vi "create harp files (main).vi"() -> ()   [LabVIEW 2010]
panel:
  in  "Close":bool
  in  "Create":bool
  in  "Create these ones?":bool
  in  "path":path
  # "Files that can be updated through this script\nwithout affecting the application code:\n - main.c\n - app.h\n - app_funcs.h\n - app_ios_and_regs.h\n - app_ios_and_regs.c"
  # "Files to give extra caution:\n - app.c\n - app_funcs.c\n - interrupts.c"
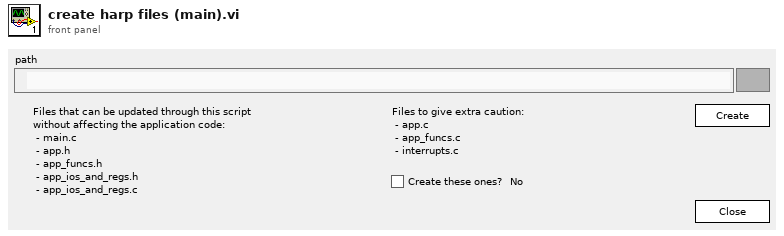
[diagram p1: front panel]
types:
  T1 = enum16{"open", "replace", "create", "open or create", "replace or create", "replace or create with confirmation"}
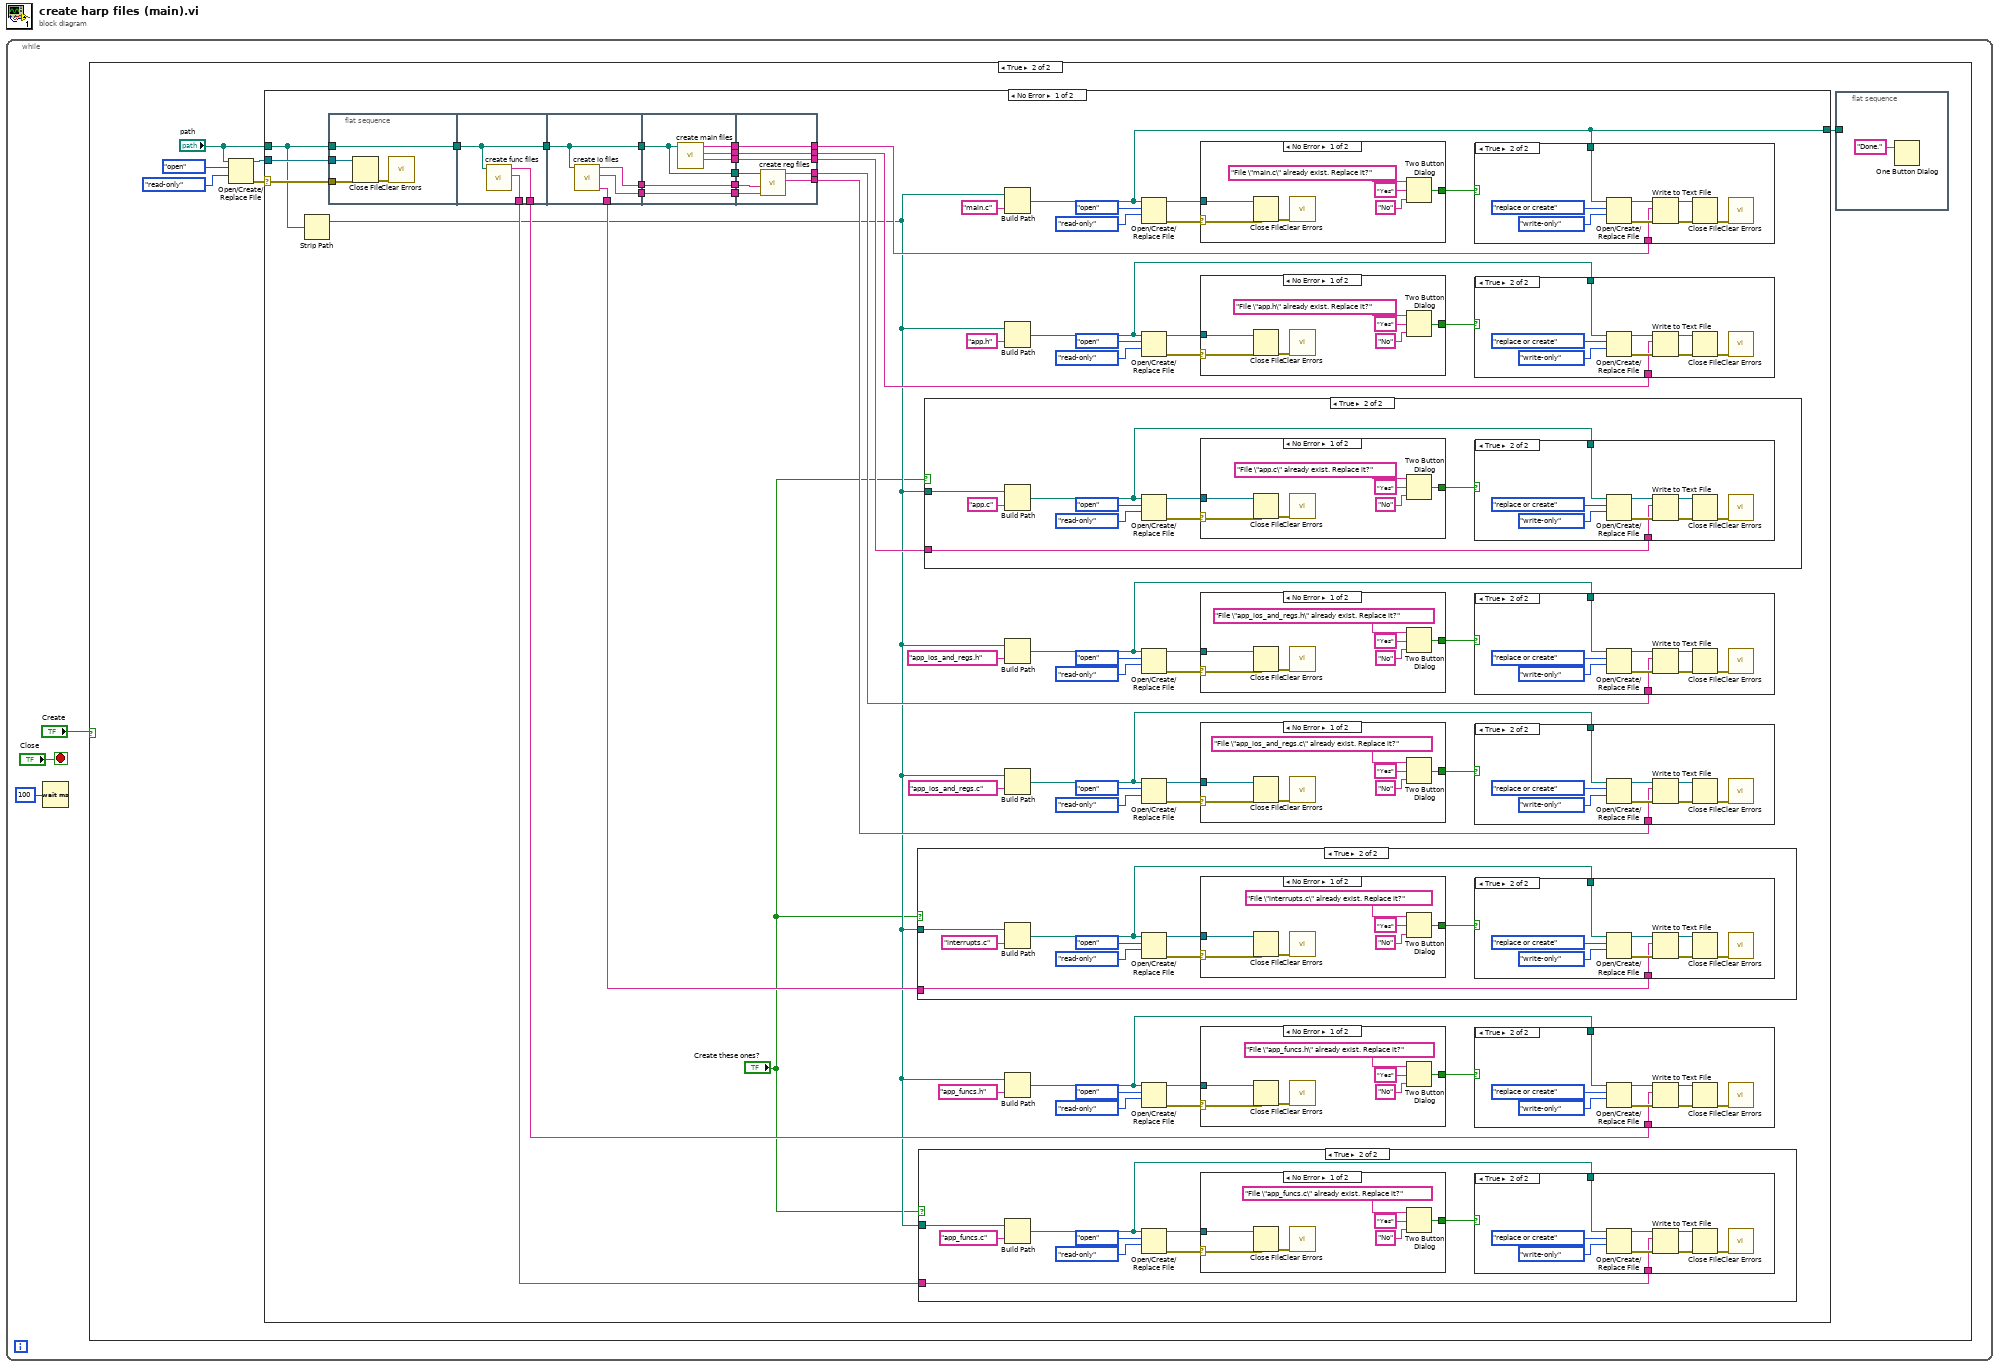
[diagram p0: block diagram]
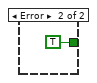
[diagram p5: hidden frame]
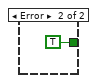
[diagram p8: hidden frame]
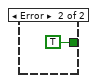
[diagram p11: hidden frame]
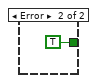
[diagram p13: hidden frame]
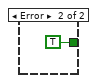
[diagram p15: hidden frame]
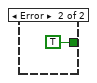
[diagram p17: hidden frame]
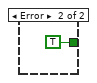
[diagram p19: hidden frame]
diagram:
  n1 = while {
    stop <- "Close" stop-if-true
    n2 = Wait (ms)(milliseconds to wait=u32 100) -> ()  [unwired: 1 out]
    n3 = case shown="True" "Create" {
      frame False {
      }
      frame True {
        n4 = Open/Create/Replace File(file path (use dialog)="path", operation (0:open)=T1."open", access (0:read/write)=enum16{"read/write", "read-only", "write-only"}."read-only") -> (refnum out=w6:refnum<file>, error out=w7:errorcluster)  [unwired: 3 in, 1 out]
        n5 = case shown="No Error" w7 {
          selector: w7 -> [w69 _]
          tunnel: w6 -> [w68 _]
          tunnel: "path" -> [w62 _]
          tunnel: [w19 _] -> w4
          frame No Error {
            n6 = Strip Path(path=w62) -> (stripped path=w20:path)  [unwired: 1 out]
            n7 = flat-sequence {
              tunnel: w69 -> [w236]
              tunnel: w68 -> [w235]
              tunnel: w62 -> [w233]
              tunnel: [w233] -> w25
              tunnel: w25 -> [w239]
              tunnel: [w239] -> w24
              tunnel: [w238] -> w23
              tunnel: [w237] -> w22
              tunnel: w24 -> [w243]
              tunnel: [w243] -> w30
              tunnel: [w242] -> w28
              tunnel: [w241] -> w26
              tunnel: [w240] -> w21
              tunnel: w30 -> [w246]
              tunnel: [w249] -> w50
              tunnel: [w248] -> w49
              tunnel: [w247] -> w48
              tunnel: [w246] -> w47
              tunnel: [w245] -> w29
              tunnel: w28 -> [w245]
              tunnel: [w244] -> w27
              tunnel: w26 -> [w244]
              tunnel: [w255] -> w51
              tunnel: [w256] -> w52
              tunnel: [w257] -> w60
              tunnel: w50 -> [w257]
              tunnel: w49 -> [w256]
              tunnel: w48 -> [w255]
              tunnel: w47 -> [w254]
              tunnel: [w253] -> w32
              tunnel: [w252] -> w31
              tunnel: w29 -> [w251]
              tunnel: w27 -> [w250]
              frame #0 {
                n8 = Close File(refnum=w235, error in=w236) -> (error out=w234:errorcluster)  [unwired: 1 out]
                n9 = call <vilib>:"Clear Errors.vi"("error in (no error)"=w234) -> ()  [unwired: 6 in, 1 out]
              }
              frame #1 {
                n10 = call "create func files.vi"("path"=w239) -> ("funtions.c"=w237:string, "funtions.h"=w238:string)  [unwired: 9 in]
              }
              frame #2 {
                n11 = call "create io files.vi"("path"=w243) -> ("interrupts.c"=w240:string, "void init_ios(void)"=w241:string, "defines"=w242:string)  [unwired: 8 in]
              }
              frame #3 {
                n12 = call "create main files.vi"("path"=w246) -> ("app.c"=w247:string, "app.h"=w248:string, "main.c"=w249:string)  [unwired: 8 in]
              }
              frame #4 {
                n13 = call "create reg files.vi"("void init_ios(void)"=w250, "defines"=w251, "path"=w254) -> ("app_regs.c"=w252:string, "app_regs.h"=w253:string)  [unwired: 7 in]
              }
            }
            n14 = case shown="True" "Create these ones?" {
              tunnel: w21 -> [_ w104]
              tunnel: w20 -> [_ w103]
              frame False {
              }
              frame True {
                n15 = Build Path(base path=w103, name or relative path="interrupts.c") -> (appended path=w98:path)
                n16 = Open/Create/Replace File(file path (use dialog)=w98, operation (0:open)=T1."open", access (0:read/write)=enum16{"read/write", "read-only", "write-only"}."read-only") -> (refnum out=w99:refnum<file>, error out=w100:errorcluster)  [unwired: 3 in, 1 out]
                n17 = case shown="No Error" w100 {
                  selector: w100 -> [w117 _]
                  tunnel: w99 -> [w116 _]
                  tunnel: [w114 TRUE ("T button?")] -> w97
                  frame No Error {
                    n18 = Close File(refnum=w116, error in=w117) -> (error out=w115:errorcluster)  [unwired: 1 out]
                    n19 = call <vilib>:"Clear Errors.vi"("error in (no error)"=w115) -> ()  [unwired: 6 in, 1 out]
                    n20 = Two Button Dialog(message="File \"interrupts.c\" already exist. Replace it?", 1:"No" ("F button name (\"Cancel\")"), 2:"Yes" ("T button name (\"OK\")")) -> (T button?=w114:bool)
                  }
                  frame Error {
                  }
                }
                n21 = case shown="True" w97 {
                  tunnel: w98 -> [_ w111]
                  tunnel: w104 -> [_ w108]
                  frame False {
                  }
                  frame True {
                    n22 = Open/Create/Replace File(file path (use dialog)=w111, operation (0:open)=T1."replace or create", access (0:read/write)=enum16{"read/write", "read-only", "write-only"}."write-only") -> (refnum out=w109:refnum<file>, error out=w110:errorcluster)  [unwired: 3 in, 1 out]
                    n23 = Write to Text File(file (use dialog)=w109, text=w108, error in=w110) -> (refnum out=w105:refnum<file>, error out=w106:errorcluster)  [unwired: 1 in, 1 out]
                    n24 = Close File(refnum=w105, error in=w106) -> (error out=w107:errorcluster)  [unwired: 1 out]
                    n25 = call <vilib>:"Clear Errors.vi"("error in (no error)"=w107) -> ()  [unwired: 6 in, 1 out]
                  }
                }
              }
            }
            n26 = case shown="True" "Create these ones?" {
              tunnel: w22 -> [_ w130]
              tunnel: w20 -> [_ w129]
              frame False {
              }
              frame True {
                n27 = Build Path(base path=w129, name or relative path="app_funcs.c") -> (appended path=w126:path)
                n28 = Open/Create/Replace File(file path (use dialog)=w126, operation (0:open)=T1."open", access (0:read/write)=enum16{"read/write", "read-only", "write-only"}."read-only") -> (refnum out=w125:refnum<file>, error out=w124:errorcluster)  [unwired: 3 in, 1 out]
                n29 = case shown="No Error" w124 {
                  selector: w124 -> [w143 _]
                  tunnel: w125 -> [w142 _]
                  tunnel: [w140 TRUE ("T button?")] -> w127
                  frame No Error {
                    n30 = Close File(refnum=w142, error in=w143) -> (error out=w141:errorcluster)  [unwired: 1 out]
                    n31 = call <vilib>:"Clear Errors.vi"("error in (no error)"=w141) -> ()  [unwired: 6 in, 1 out]
                    n32 = Two Button Dialog(message="File \"app_funcs.c\" already exist. Replace it?", 1:"No" ("F button name (\"Cancel\")"), 2:"Yes" ("T button name (\"OK\")")) -> (T button?=w140:bool)
                  }
                  frame Error {
                  }
                }
                n33 = case shown="True" w127 {
                  tunnel: w126 -> [_ w137]
                  tunnel: w130 -> [_ w134]
                  frame False {
                  }
                  frame True {
                    n34 = Open/Create/Replace File(file path (use dialog)=w137, operation (0:open)=T1."replace or create", access (0:read/write)=enum16{"read/write", "read-only", "write-only"}."write-only") -> (refnum out=w135:refnum<file>, error out=w136:errorcluster)  [unwired: 3 in, 1 out]
                    n35 = Write to Text File(file (use dialog)=w135, text=w134, error in=w136) -> (refnum out=w131:refnum<file>, error out=w132:errorcluster)  [unwired: 1 in, 1 out]
                    n36 = Close File(refnum=w131, error in=w132) -> (error out=w133:errorcluster)  [unwired: 1 out]
                    n37 = call <vilib>:"Clear Errors.vi"("error in (no error)"=w133) -> ()  [unwired: 6 in, 1 out]
                  }
                }
              }
            }
            n38 = case shown="True" "Create these ones?" {
              tunnel: w51 -> [_ w71]
              tunnel: w20 -> [_ w70]
              frame False {
              }
              frame True {
                n39 = Build Path(base path=w70, name or relative path="app.c") -> (appended path=w74:path)
                n40 = Open/Create/Replace File(file path (use dialog)=w74, operation (0:open)=T1."open", access (0:read/write)=enum16{"read/write", "read-only", "write-only"}."read-only") -> (refnum out=w75:refnum<file>, error out=w76:errorcluster)  [unwired: 3 in, 1 out]
                n41 = case shown="No Error" w76 {
                  selector: w76 -> [w91 _]
                  tunnel: w75 -> [w90 _]
                  tunnel: [w88 TRUE ("T button?")] -> w73
                  frame No Error {
                    n42 = Close File(refnum=w90, error in=w91) -> (error out=w89:errorcluster)  [unwired: 1 out]
                    n43 = call <vilib>:"Clear Errors.vi"("error in (no error)"=w89) -> ()  [unwired: 6 in, 1 out]
                    n44 = Two Button Dialog(message="File \"app.c\" already exist. Replace it?", 1:"No" ("F button name (\"Cancel\")"), 2:"Yes" ("T button name (\"OK\")")) -> (T button?=w88:bool)
                  }
                  frame Error {
                  }
                }
                n45 = case shown="True" w73 {
                  tunnel: w74 -> [_ w85]
                  tunnel: w71 -> [_ w82]
                  frame False {
                  }
                  frame True {
                    n46 = Open/Create/Replace File(file path (use dialog)=w85, operation (0:open)=T1."replace or create", access (0:read/write)=enum16{"read/write", "read-only", "write-only"}."write-only") -> (refnum out=w83:refnum<file>, error out=w84:errorcluster)  [unwired: 3 in, 1 out]
                    n47 = Write to Text File(file (use dialog)=w83, text=w82, error in=w84) -> (refnum out=w79:refnum<file>, error out=w80:errorcluster)  [unwired: 1 in, 1 out]
                    n48 = Close File(refnum=w79, error in=w80) -> (error out=w81:errorcluster)  [unwired: 1 out]
                    n49 = call <vilib>:"Clear Errors.vi"("error in (no error)"=w81) -> ()  [unwired: 6 in, 1 out]
                  }
                }
              }
            }
            n50 = Build Path(base path=w20, name or relative path="main.c") -> (appended path=w19:path)
            n51 = Build Path(base path=w20, name or relative path="app.h") -> (appended path=w57:path)
            n52 = Build Path(base path=w20, name or relative path="app_ios_and_regs.h") -> (appended path=w37:path)
            n53 = Build Path(base path=w20, name or relative path="app_ios_and_regs.c") -> (appended path=w42:path)
            n54 = Build Path(base path=w20, name or relative path="app_funcs.h") -> (appended path=w14:path)
            n55 = Open/Create/Replace File(file path (use dialog)=w19, operation (0:open)=T1."open", access (0:read/write)=enum16{"read/write", "read-only", "write-only"}."read-only") -> (refnum out=w64:refnum<file>, error out=w65:errorcluster)  [unwired: 3 in, 1 out]
            n56 = Open/Create/Replace File(file path (use dialog)=w57, operation (0:open)=T1."open", access (0:read/write)=enum16{"read/write", "read-only", "write-only"}."read-only") -> (refnum out=w56:refnum<file>, error out=w55:errorcluster)  [unwired: 3 in, 1 out]
            n57 = Open/Create/Replace File(file path (use dialog)=w37, operation (0:open)=T1."open", access (0:read/write)=enum16{"read/write", "read-only", "write-only"}."read-only") -> (refnum out=w36:refnum<file>, error out=w35:errorcluster)  [unwired: 3 in, 1 out]
            n58 = Open/Create/Replace File(file path (use dialog)=w42, operation (0:open)=T1."open", access (0:read/write)=enum16{"read/write", "read-only", "write-only"}."read-only") -> (refnum out=w43:refnum<file>, error out=w44:errorcluster)  [unwired: 3 in, 1 out]
            n59 = Open/Create/Replace File(file path (use dialog)=w14, operation (0:open)=T1."open", access (0:read/write)=enum16{"read/write", "read-only", "write-only"}."read-only") -> (refnum out=w15:refnum<file>, error out=w16:errorcluster)  [unwired: 3 in, 1 out]
            n60 = case shown="No Error" w65 {
              selector: w65 -> [w228 _]
              tunnel: w64 -> [w227 _]
              tunnel: [w225 TRUE ("T button?")] -> w63
              frame No Error {
                n61 = Close File(refnum=w227, error in=w228) -> (error out=w226:errorcluster)  [unwired: 1 out]
                n62 = call <vilib>:"Clear Errors.vi"("error in (no error)"=w226) -> ()  [unwired: 6 in, 1 out]
                n63 = Two Button Dialog(message="File \"main.c\" already exist. Replace it?", 1:"No" ("F button name (\"Cancel\")"), 2:"Yes" ("T button name (\"OK\")")) -> (T button?=w225:bool)
              }
              frame Error {
              }
            }
            n64 = case shown="No Error" w55 {
              selector: w55 -> [w211 _]
              tunnel: w56 -> [w210 _]
              tunnel: [w208 TRUE ("T button?")] -> w58
              frame No Error {
                n65 = Close File(refnum=w210, error in=w211) -> (error out=w209:errorcluster)  [unwired: 1 out]
                n66 = call <vilib>:"Clear Errors.vi"("error in (no error)"=w209) -> ()  [unwired: 6 in, 1 out]
                n67 = Two Button Dialog(message="File \"app.h\" already exist. Replace it?", 1:"No" ("F button name (\"Cancel\")"), 2:"Yes" ("T button name (\"OK\")")) -> (T button?=w208:bool)
              }
              frame Error {
              }
            }
            n68 = case shown="No Error" w35 {
              selector: w35 -> [w194 _]
              tunnel: w36 -> [w193 _]
              tunnel: [w191 TRUE ("T button?")] -> w38
              frame No Error {
                n69 = Close File(refnum=w193, error in=w194) -> (error out=w192:errorcluster)  [unwired: 1 out]
                n70 = call <vilib>:"Clear Errors.vi"("error in (no error)"=w192) -> ()  [unwired: 6 in, 1 out]
                n71 = Two Button Dialog(message="File \"app_ios_and_regs.h\" already exist. Replace it?", 1:"No" ("F button name (\"Cancel\")"), 2:"Yes" ("T button name (\"OK\")")) -> (T button?=w191:bool)
              }
              frame Error {
              }
            }
            n72 = case shown="No Error" w44 {
              selector: w44 -> [w177 _]
              tunnel: w43 -> [w176 _]
              tunnel: [w174 TRUE ("T button?")] -> w41
              frame No Error {
                n73 = Close File(refnum=w176, error in=w177) -> (error out=w175:errorcluster)  [unwired: 1 out]
                n74 = call <vilib>:"Clear Errors.vi"("error in (no error)"=w175) -> ()  [unwired: 6 in, 1 out]
                n75 = Two Button Dialog(message="File \"app_ios_and_regs.c\" already exist. Replace it?", 1:"No" ("F button name (\"Cancel\")"), 2:"Yes" ("T button name (\"OK\")")) -> (T button?=w174:bool)
              }
              frame Error {
              }
            }
            n76 = case shown="No Error" w16 {
              selector: w16 -> [w160 _]
              tunnel: w15 -> [w159 _]
              tunnel: [w157 TRUE ("T button?")] -> w13
              frame No Error {
                n77 = Close File(refnum=w159, error in=w160) -> (error out=w158:errorcluster)  [unwired: 1 out]
                n78 = call <vilib>:"Clear Errors.vi"("error in (no error)"=w158) -> ()  [unwired: 6 in, 1 out]
                n79 = Two Button Dialog(message="File \"app_funcs.h\" already exist. Replace it?", 1:"No" ("F button name (\"Cancel\")"), 2:"Yes" ("T button name (\"OK\")")) -> (T button?=w157:bool)
              }
              frame Error {
              }
            }
            n80 = case shown="True" w63 {
              tunnel: w19 -> [_ w222]
              tunnel: w60 -> [_ w219]
              frame False {
              }
              frame True {
                n81 = Open/Create/Replace File(file path (use dialog)=w222, operation (0:open)=T1."replace or create", access (0:read/write)=enum16{"read/write", "read-only", "write-only"}."write-only") -> (refnum out=w220:refnum<file>, error out=w221:errorcluster)  [unwired: 3 in, 1 out]
                n82 = Write to Text File(file (use dialog)=w220, text=w219, error in=w221) -> (refnum out=w216:refnum<file>, error out=w217:errorcluster)  [unwired: 1 in, 1 out]
                n83 = Close File(refnum=w216, error in=w217) -> (error out=w218:errorcluster)  [unwired: 1 out]
                n84 = call <vilib>:"Clear Errors.vi"("error in (no error)"=w218) -> ()  [unwired: 6 in, 1 out]
              }
            }
            n85 = case shown="True" w58 {
              tunnel: w57 -> [_ w205]
              tunnel: w52 -> [_ w202]
              frame False {
              }
              frame True {
                n86 = Open/Create/Replace File(file path (use dialog)=w205, operation (0:open)=T1."replace or create", access (0:read/write)=enum16{"read/write", "read-only", "write-only"}."write-only") -> (refnum out=w203:refnum<file>, error out=w204:errorcluster)  [unwired: 3 in, 1 out]
                n87 = Write to Text File(file (use dialog)=w203, text=w202, error in=w204) -> (refnum out=w199:refnum<file>, error out=w200:errorcluster)  [unwired: 1 in, 1 out]
                n88 = Close File(refnum=w199, error in=w200) -> (error out=w201:errorcluster)  [unwired: 1 out]
                n89 = call <vilib>:"Clear Errors.vi"("error in (no error)"=w201) -> ()  [unwired: 6 in, 1 out]
              }
            }
            n90 = case shown="True" w38 {
              tunnel: w37 -> [_ w188]
              tunnel: w32 -> [_ w185]
              frame False {
              }
              frame True {
                n91 = Open/Create/Replace File(file path (use dialog)=w188, operation (0:open)=T1."replace or create", access (0:read/write)=enum16{"read/write", "read-only", "write-only"}."write-only") -> (refnum out=w186:refnum<file>, error out=w187:errorcluster)  [unwired: 3 in, 1 out]
                n92 = Write to Text File(file (use dialog)=w186, text=w185, error in=w187) -> (refnum out=w182:refnum<file>, error out=w183:errorcluster)  [unwired: 1 in, 1 out]
                n93 = Close File(refnum=w182, error in=w183) -> (error out=w184:errorcluster)  [unwired: 1 out]
                n94 = call <vilib>:"Clear Errors.vi"("error in (no error)"=w184) -> ()  [unwired: 6 in, 1 out]
              }
            }
            n95 = case shown="True" w41 {
              tunnel: w42 -> [_ w171]
              tunnel: w31 -> [_ w168]
              frame False {
              }
              frame True {
                n96 = Open/Create/Replace File(file path (use dialog)=w171, operation (0:open)=T1."replace or create", access (0:read/write)=enum16{"read/write", "read-only", "write-only"}."write-only") -> (refnum out=w169:refnum<file>, error out=w170:errorcluster)  [unwired: 3 in, 1 out]
                n97 = Write to Text File(file (use dialog)=w169, text=w168, error in=w170) -> (refnum out=w165:refnum<file>, error out=w166:errorcluster)  [unwired: 1 in, 1 out]
                n98 = Close File(refnum=w165, error in=w166) -> (error out=w167:errorcluster)  [unwired: 1 out]
                n99 = call <vilib>:"Clear Errors.vi"("error in (no error)"=w167) -> ()  [unwired: 6 in, 1 out]
              }
            }
            n100 = case shown="True" w13 {
              tunnel: w14 -> [_ w154]
              tunnel: w23 -> [_ w151]
              frame False {
              }
              frame True {
                n101 = Open/Create/Replace File(file path (use dialog)=w154, operation (0:open)=T1."replace or create", access (0:read/write)=enum16{"read/write", "read-only", "write-only"}."write-only") -> (refnum out=w152:refnum<file>, error out=w153:errorcluster)  [unwired: 3 in, 1 out]
                n102 = Write to Text File(file (use dialog)=w152, text=w151, error in=w153) -> (refnum out=w148:refnum<file>, error out=w149:errorcluster)  [unwired: 1 in, 1 out]
                n103 = Close File(refnum=w148, error in=w149) -> (error out=w150:errorcluster)  [unwired: 1 out]
                n104 = call <vilib>:"Clear Errors.vi"("error in (no error)"=w150) -> ()  [unwired: 6 in, 1 out]
              }
            }
          }
          frame Error {
            n105 = One Button Dialog(message="Error: Selected file doesn't exist.") -> ()  [unwired: 1 in, 1 out]
          }
        }
        n106 = flat-sequence {
          tunnel: w4 -> [_]
          frame #0 {
            n107 = One Button Dialog(message="Done.") -> ()  [unwired: 1 in, 1 out]
          }
        }
      }
    }
  }
